vi "NI5112.get scan status.vi"(0 "i ref in":refnum<vi>, 3 "ms timeout (100)":i32=100, 5 "error in (no error)":errorcluster) -> (14 "i ref out":refnum<vi>, 16 "x != y?":bool, 17 "timed out":bool, 19 "error out":errorcluster)   [LabVIEW 2014, in "NI5112.lvlib"]
uses:
  NI5112.lvlib
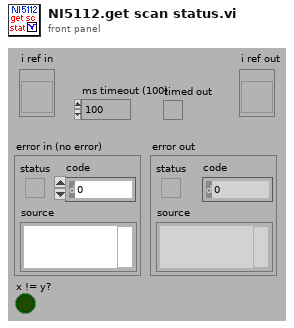
[diagram p1: front panel]
types:
  T1 = typedef "NI5112.lvlib/NI5112.i attribute.ctl" = cluster{"HWChannel":string, "instrument handle":refnum<k15>, "BinWidth":dbl, "vertical offset":dbl, "vertical range":dbl, "DataBPR":i32, "5112BPR":i32, "FullSpeed":bool, "discrLevel":dbl, "DoDiscr":bool, "VerCoupling":string}
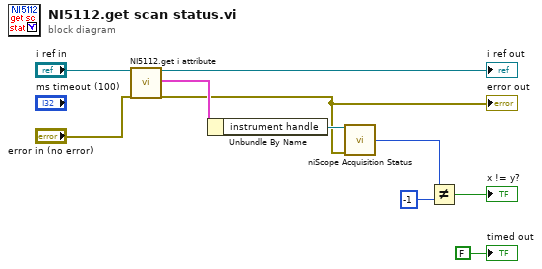
[diagram p0: block diagram]
diagram:
  n1 = call "NI5112.get i attribute.vi"("i ref in"="i ref in", "error in (no error)"="error in (no error)") -> ("i ref out"=→"i ref out":refnum<vi>, "i attribute"=w8:T1, "error out"=w3:errorcluster)  [unwired: 15 in]
  "error out" <- w3
  n2 = Unbundle By Name(w8) -> ("instrument handle"=w6:refnum<k15>)
  n3 = call <instrlib>:"niScope Acquisition Status.vi"("instrument handle"=w6, "error in"=w3) -> ("acquisition status"=w5:i32)  [unwired: 11 in, 2 out]
  n4 = Not Equal?(x=w5, y=-1) -> (x != y?=→"x != y?":bool)
  "timed out" <- FALSE ("timed out")
